vi "Get Marker Present.vi"(8 "error in (no error)":errorcluster, 11 "Mouse in":refnum<class "Mouse.lvclass">) -> (0 "error out":errorcluster, 2 "Marker":bool, 3 "Mouse out":refnum<class "Mouse.lvclass">)   [LabVIEW 2020, in "Maze.lvlib" / "Mouse.lvclass"]
uses:
  Mouse.lvclass
  Mouse.lvclass/Mouse.ctl
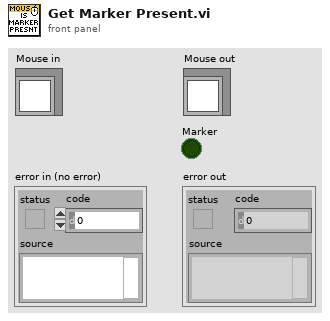
[diagram p1: front panel]
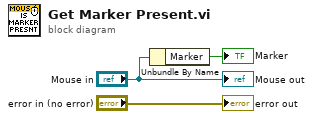
[diagram p0: block diagram]
diagram:
  n1 = Unbundle By Name("Mouse in") -> ("Marker"=→"Marker":bool)
  "error out" <- "error in (no error)"
  "Mouse out" <- "Mouse in"
